vi "host.vi"() -> ()   [LabVIEW 2018]
uses:
  <vilib>/userdefined/High Color/nirio_resource_hc.ctl
  <instrlib>/niDCPower/nidcpower.llb/niDCPower Measurement Type.ctl
  <vilib>/FPGAPlugInAG/PXI-7953R/niLvFpga_Open_PXI-7953R.vi
  <vilib>/rvi/interface/common/dynamic/niFpgaDynamicAddResources.vi
  <vilib>/Utility/error.llb/Error Cluster From Error Code.vi
  <vilib>/rvi/errors/niLvFpgaAdjustHostInterfaceError.vi
  <vilib>/FPGAPlugInAG/Dynamic/niLvFpga_Close_Dynamic.vi
  <vilib>/rvi/interface/nirviOpenFPGA/nirviOpenFPGA.xnode
  FPGA Bitfiles/displayproj_FPGATarget_target_ybt1itgLS5Q.lvbitx
  <vilib>/rvi/interface/nirviReadWriteControl/nirviReadWriteControl.xnode
  <vilib>/rvi/interface/nirviCloseFPGA/nirviCloseFPGA.xnode
  NiFpgaLv.dll
  <vilib>/rvi/interface/Simulation/niFpgaSimulationCallBeginRW.vi
panel:
  out "LOS":bool
  out "FAULT":bool
  out "RX_DV/LOS":bool
  out "RX_ER/PRBS_PASS":bool
  in  "125MHZ_OE":bool
  in  "LOOPEN":bool
  in  "ENABLE":bool
  in  "LCKREFN":bool
  in  "PRBSEN":bool
  in  "Data":u8=24 format="%x"
  out "Array":bool[](array[boolean])=[FALSE, FALSE, FALSE, TRUE, FALSE, FALSE, FALSE, FALSE]
  out "IndxReadData":i32[](array[numeric])=[22, 24, 26, 28, 30, 32, 34, 36]
  in  "WRITE":bool
  out "DETECT":bool=TRUE
  in  "counterLowFreq":i32=120
  out "SDA_READED":u64=34637845889023
  out "size(s)":i32=46
  out "ACK_BOOL 2":bool=TRUE
  out "ACK_BOOL":bool=TRUE
  out "ACK 2":i32=41
  out "ACK":i32=23
  in  "TEST_EEPROM":bool=TRUE
  out "SPI_READY":bool=TRUE
  out "Vdd_Voltage, V 2":dbl=0.0007584113885058215 caption="V" format="%_3g"
  out "Vdd_Current, mA 2":dbl=-0.0058870491630167495 caption="mA" format="%_2g"
  in  "output enabled 2":bool caption="output enabled"
  in  "output enabled":bool
  out "Vdd_Current, mA":dbl=0.00018186713296160315 caption="mA" format="%_2g"
  out "Vdd_Voltage, V":dbl=-0.00013918231455023835 caption="V" format="%_3g"
  in  "Vdd":refnum<k15>="PXI1Slot2"
  in  "Tab Control":enum32{"Чтение EEPROM", "Проверка EEPROM"}(tab)=enum."Проверка EEPROM"
  in  "EEPROM_writePath":path caption="Путь для записи EEPROM"
  in  "EEPROM_checkPath":path caption="Путь для проверки EEPROM"
  out "REG_ERROR":i32
  out "Error List":string
  in  "FPGA name":T1="PXI1Slot5" caption="RIO Device"
  in  "Start":bool
  in  "Comand":bool
  in  "stop":bool=TRUE
  # "Ch2"
  # "Ch1"
  # "Запись/Чтение"
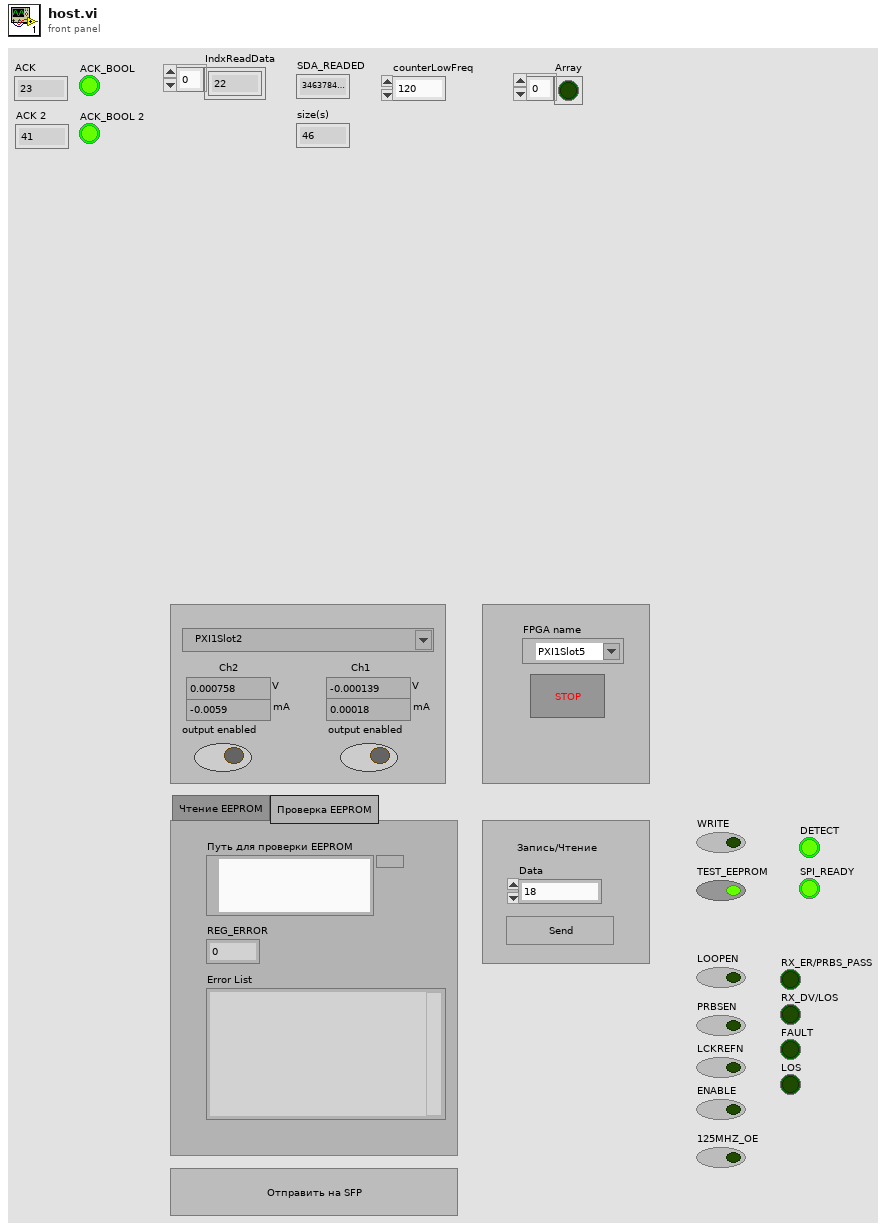
[diagram p1: front panel]
types:
  T1 = typedef "nirio_resource_hc.ctl" = tag
  T2 = enum16{"open", "replace", "create", "open or create", "replace or create", "replace or create with confirmation"}
  T3 = typedef "niDCPower Measurement Type.ctl" = i32
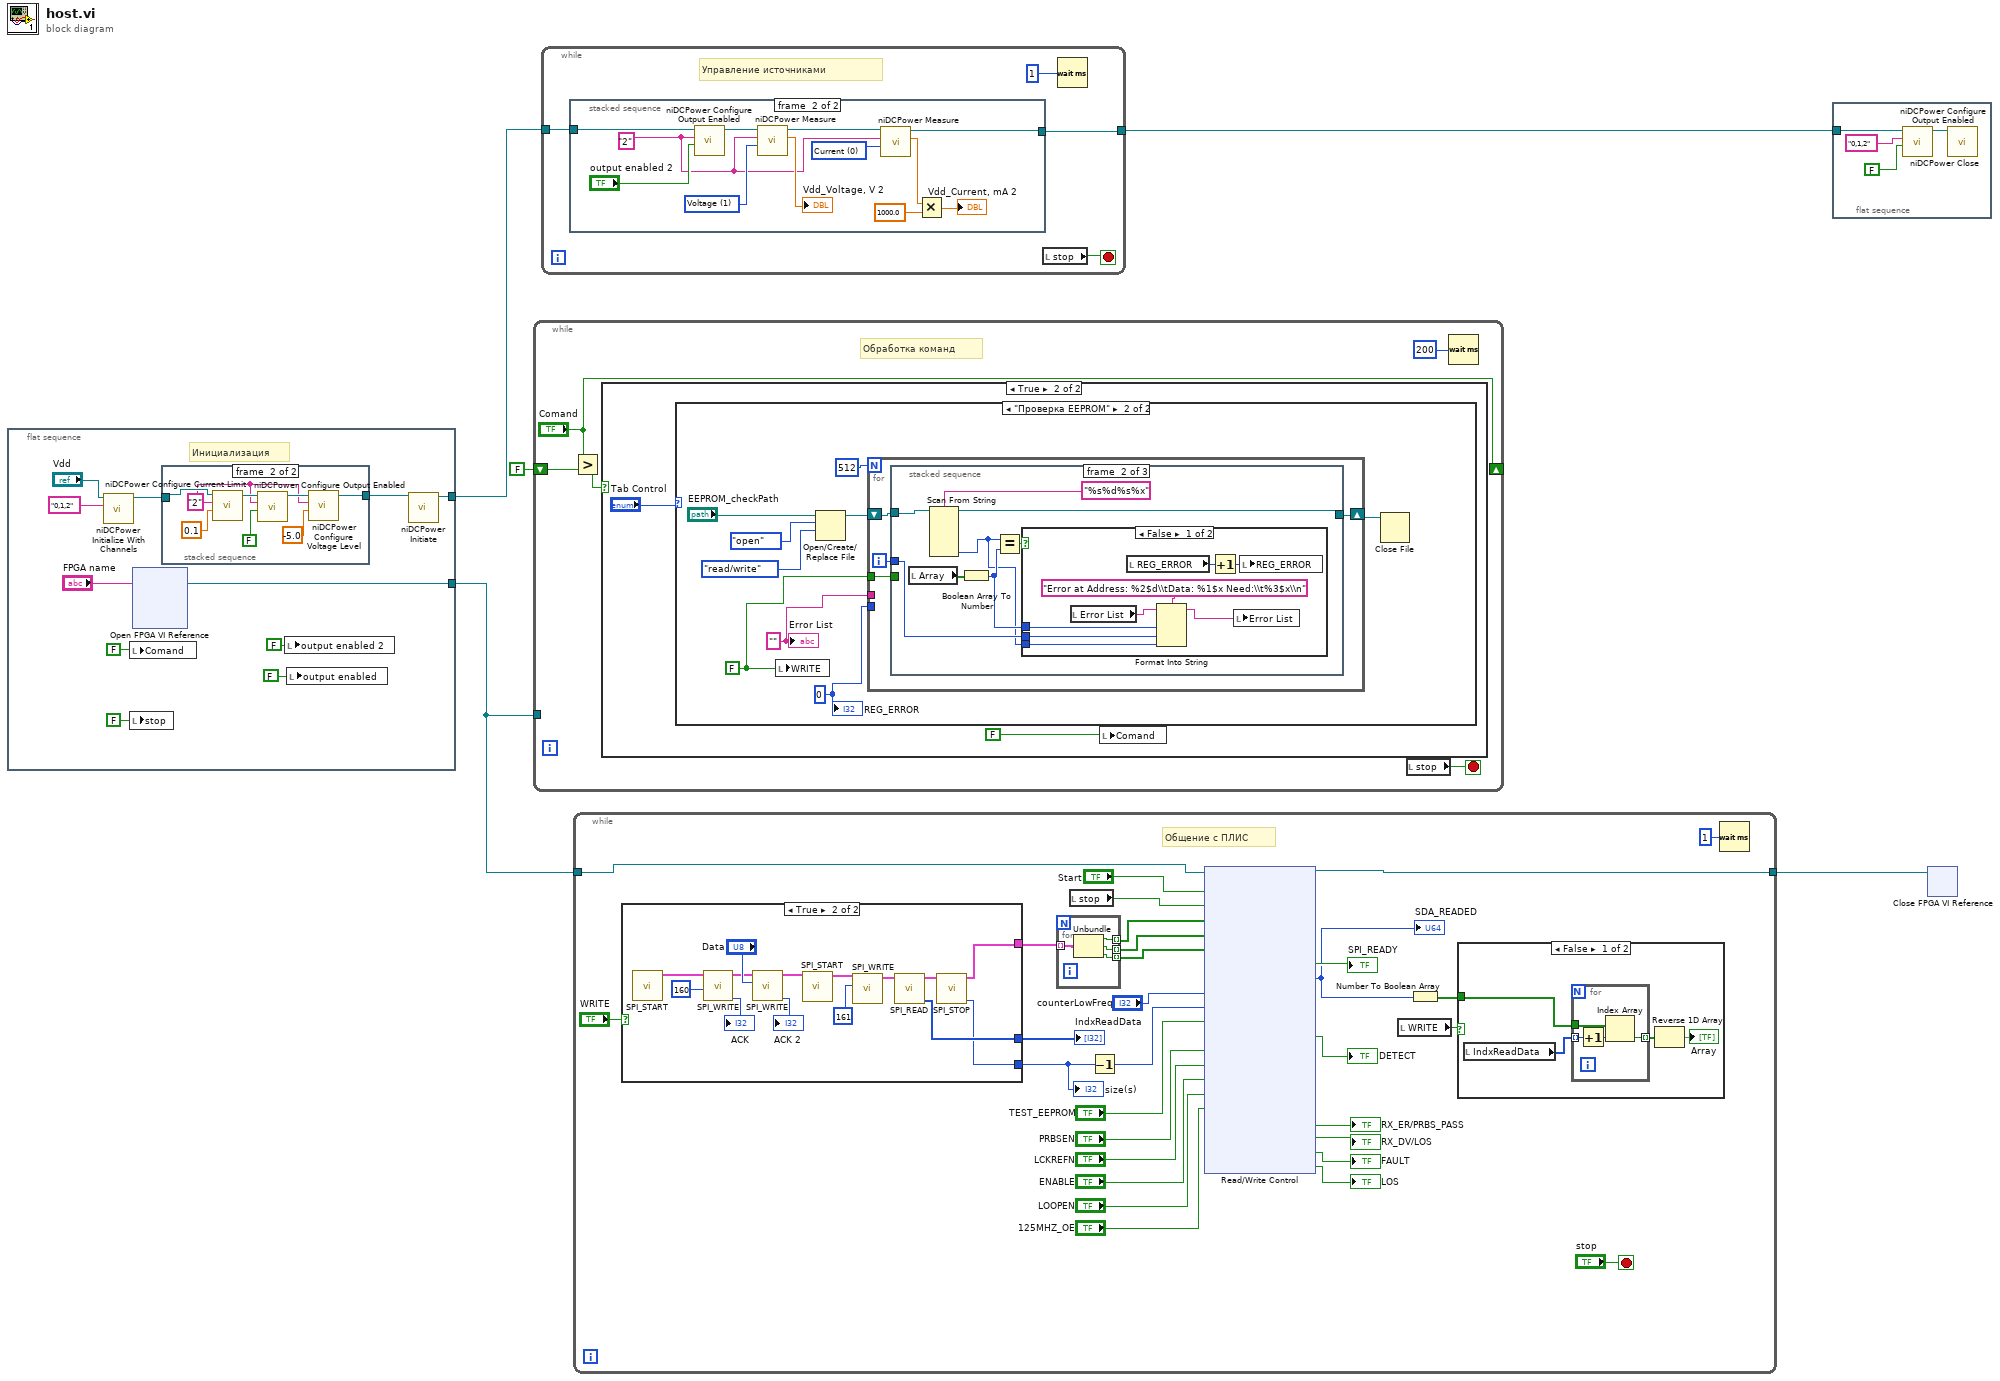
[diagram p0: block diagram]
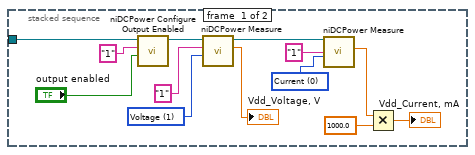
[diagram p2: hidden frame]
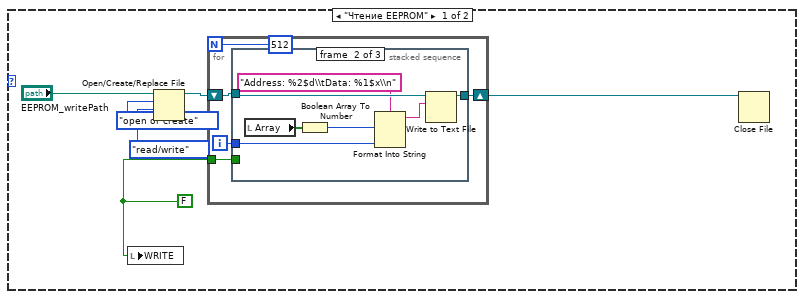
[diagram p4: hidden frame]
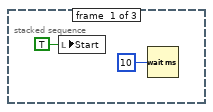
[diagram p5: hidden frame]
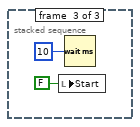
[diagram p6: hidden frame]
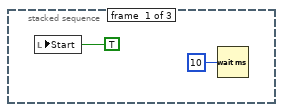
[diagram p7: hidden frame]
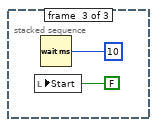
[diagram p9: hidden frame]
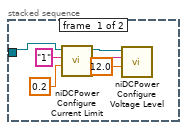
[diagram p10: hidden frame]
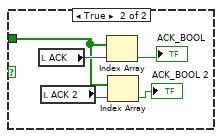
[diagram p11: hidden frame]
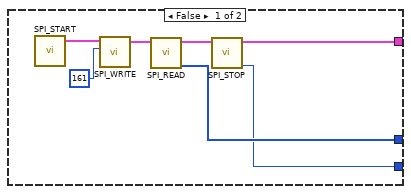
[diagram p12: hidden frame]
diagram:
  n1 = flat-sequence {
    tunnel: [w16] -> w4
    tunnel: [w8] -> w2
    frame #0 {
      # "Инициализация"
      n2 = call <instrlib>:"niDCPower Initialize With Channels.vi"("channels"="0,1,2", "resource name"="Vdd") -> ("instrument handle out"=w10:refnum<k15>)  [unwired: 8 in, 1 out]
      n3 = local write "Comand"(FALSE ("Comand")) -> ()
      n4 = local write "stop"(FALSE ("stop")) -> ()
      n5 = xnode "Open FPGA VI Reference"("resource name"="FPGA name") -> ("FPGA VI Reference Out"=w16:refnum<k20>)  [unwired: 1 in, 1 out]
      n6 = stacked-sequence {
        tunnel: [_ w27] -> w11
        tunnel: w10 -> [w20 w28]
        frame #0 {
          w18 = "1" ("channel name")
          n7 = call <instrlib>:"niDCPower Configure Current Limit.vi"("current limit"=0.2 ("current limit Vdd"), "channel name"=w18, "instrument handle"=w20) -> ("instrument handle out"=w19:refnum<k15>)  [unwired: 7 in, 1 out]
          n8 = call <instrlib>:"niDCPower Configure Voltage Level.vi"("voltage level"=12.0, "channel name"=w18, "instrument handle"=w19) -> ()  [unwired: 7 in, 2 out]
        }
        frame #1 {
          w24 = "2" ("channel name")
          n9 = call <instrlib>:"niDCPower Configure Current Limit.vi"("current limit"=0.1 ("current limit Vdd"), "channel name"=w24, "instrument handle"=w28) -> ("instrument handle out"=w25:refnum<k15>)  [unwired: 7 in, 1 out]
          n10 = call <instrlib>:"niDCPower Configure Output Enabled.vi"("output enabled"=FALSE, "channel name"=w24, "instrument handle"=w25) -> ("instrument handle out"=w26:refnum<k15>)  [unwired: 7 in, 1 out]
          n11 = call <instrlib>:"niDCPower Configure Voltage Level.vi"("voltage level"=-5.0, "channel name"=w24, "instrument handle"=w26) -> ("instrument handle out"=w27:refnum<k15>)  [unwired: 7 in, 1 out]
        }
      }
      n12 = local write "output enabled 2"(FALSE ("output enabled")) -> ()
      n13 = local write "output enabled"(FALSE ("output enabled")) -> ()
      n14 = call <instrlib>:"niDCPower Initiate.vi"("instrument handle"=w11) -> ("instrument handle out"=w8:refnum<k15>)  [unwired: 9 in, 1 out]
    }
  }
  n15 = while {
    tunnel: w4 -> [_]
    shift-right: ["Comand"] -> _
    shift-left: FALSE ("Comand") -> [w30]
    stop <- w34 stop-if-true
    # "Обработка команд"
    n16 = Greater?(x="Comand", y=w30) -> (0:w32:bool)
    n17 = case shown="True" w32 {
      frame False {
      }
      frame True {
        n18 = case shown="\"Проверка EEPROM\"" "Tab Control" {
          frame "Чтение EEPROM" {
            w38 = FALSE ("WRITE")
            n19 = local write "WRITE"(w38) -> ()
            n20 = Open/Create/Replace File(file path (use dialog)="EEPROM_writePath", operation (0:open)=T2."open or create", access (0:read/write)=enum16{"read/write", "read-only", "write-only"}."read/write") -> (refnum out=w40:refnum<file>)  [unwired: 3 in, 2 out]
            n21 = for {
              N: 512 -> [_]
              tunnel: w38 -> [w45]
              shift-right: [w46] -> w39
              shift-left: w40 -> [w47]
              i -> [w44]
              n22 = stacked-sequence {
                tunnel: w47 -> [_ w56 _]
                tunnel: [_ w55 _] -> w46
                tunnel: w45 -> [_ _ _]
                tunnel: w44 -> [_ w52 _]
                frame #0 {
                  n23 = local write "Start"(TRUE ("Start")) -> ()
                  n24 = Wait (ms)(milliseconds to wait=u32 10) -> ()  [unwired: 1 out]
                }
                frame #1 {
                  n25 = local read "Array"() -> (w54:bool[])
                  n26 = Boolean Array To Number(Boolean array=w54) -> (number=w53:u32)
                  n27 = Format Into String(format string="Address: %2$d\\tData: %1$x\\n", w53, w52) -> (resulting string=w51:string)  [unwired: 2 in, 1 out]
                  n28 = Write to Text File(file (use dialog)=w56, text=w51) -> (refnum out=w55:refnum<file>)  [unwired: 2 in, 2 out]
                }
                frame #2 {
                  n29 = local write "Start"(FALSE ("Start")) -> ()
                  n30 = Wait (ms)(milliseconds to wait=u32 10) -> ()  [unwired: 1 out]
                }
              }
            }
            n31 = Close File(refnum=w39) -> ()  [unwired: 1 in, 2 out]
          }
          frame "Проверка EEPROM" {
            w59 = "" ("String")
            w60 = 0 ("REG_ERROR")
            w62 = FALSE ("WRITE")
            n32 = local write "WRITE"(w62) -> ()
            n33 = Open/Create/Replace File(file path (use dialog)="EEPROM_checkPath", operation (0:open)=T2."open", access (0:read/write)=enum16{"read/write", "read-only", "write-only"}."read/write") -> (refnum out=w64:refnum<file>)  [unwired: 3 in, 2 out]
            n34 = for {
              N: 512 -> [_]
              tunnel: w62 -> [w69]
              shift-right: [w70] -> w63
              shift-left: w64 -> [w71]
              tunnel: w60 -> [_]
              tunnel: w59 -> [_]
              i -> [w68]
              n35 = stacked-sequence {
                tunnel: w71 -> [_ w79 _]
                tunnel: [_ w78 _] -> w70
                tunnel: w69 -> [_ _ _]
                tunnel: w68 -> [_ w75 _]
                frame #0 {
                  n36 = local write "Start"(TRUE ("Start")) -> ()
                  n37 = Wait (ms)(milliseconds to wait=u32 10) -> ()  [unwired: 1 out]
                }
                frame #1 {
                  n38 = local read "Array"() -> (w81:bool[])
                  n39 = Scan From String("%s%d%s%x" ("format string"), w79) -> (w78:refnum<file>, output 4=w74:u32)  [unwired: 8 in, 1 out]
                  n40 = Boolean Array To Number(Boolean array=w81) -> (number=w76:u32)
                  n41 = Equal?(x=w74, y=w76) -> (x = y?=w77:bool)
                  n42 = case shown="False" w77 {
                    tunnel: w76 -> [w87 _]
                    tunnel: w75 -> [w86 _]
                    tunnel: w74 -> [w82 _]
                    frame False {
                      n43 = local read "Error List"() -> (w83:string)
                      n44 = local read "REG_ERROR"() -> (w89:i32)
                      n45 = Format Into String(format string="Error at Address: %2$d\\tData: %1$x Need:\\t%3$x\\n", initial string=w83, w87, w86, w82) -> (resulting string=w84:string)  [unwired: 1 in, 1 out]
                      n46 = Increment(x=w89) -> (x+1=w88:i32)
                      n47 = local write "Error List"(w84) -> ()
                      n48 = local write "REG_ERROR"(w88) -> ()
                    }
                    frame True {
                    }
                  }
                }
                frame #2 {
                  n49 = local write "Start"(FALSE ("Start")) -> ()
                  n50 = Wait (ms)(milliseconds to wait=u32 10) -> ()  [unwired: 1 out]
                }
              }
            }
            n51 = Close File(refnum=w63) -> ()  [unwired: 1 in, 2 out]
            "REG_ERROR" <- w60
            "Error List" <- w59
          }
        }
        n52 = local write "Comand"(FALSE ("Comand")) -> ()
      }
    }
    n53 = local read "stop"() -> (w34:bool)
    n54 = Wait (ms)(milliseconds to wait=u32 200) -> ()  [unwired: 1 out]
  }
  n55 = while {
    tunnel: [w92] -> w3
    tunnel: w2 -> [w94]
    stop <- w95 stop-if-true
    # "Управление источниками"
    n56 = stacked-sequence {
      tunnel: w94 -> [w96 w111]
      tunnel: [_ w109] -> w92
      frame #0 {
        w103 = T3 0 items=["Current", "Voltage"] ("measurement type")
        w101 = T3 1 items=["Current", "Voltage"] ("measurement type")
        n57 = call <instrlib>:"niDCPower Configure Output Enabled.vi"("output enabled"="output enabled", "channel name"="1", "instrument handle"=w96) -> ("instrument handle out"=w105:refnum<k15>)  [unwired: 7 in, 1 out]
        n58 = call <instrlib>:"niDCPower Measure.vi"("measurement type"=w101, "channel name"="1", "instrument handle"=w105) -> ("measurement"=→"Vdd_Voltage, V":dbl, "instrument handle out"=w106:refnum<k15>)  [unwired: 6 in, 1 out]
        n59 = call <instrlib>:"niDCPower Measure.vi"("measurement type"=w103, "channel name"="1", "instrument handle"=w106) -> ("measurement"=w107:dbl)  [unwired: 6 in, 2 out]
        n60 = Multiply(x=w107, y=1000.0) -> (x*y=→"Vdd_Current, mA":dbl)
      }
      frame #1 {
        w116 = T3 0 items=["Current", "Voltage"] ("measurement type")
        w115 = T3 1 items=["Current", "Voltage"] ("measurement type")
        w110 = "2" ("channel name")
        n61 = call <instrlib>:"niDCPower Configure Output Enabled.vi"("output enabled"="output enabled 2", "channel name"=w110, "instrument handle"=w111) -> ("instrument handle out"=w117:refnum<k15>)  [unwired: 7 in, 1 out]
        n62 = call <instrlib>:"niDCPower Measure.vi"("measurement type"=w115, "channel name"=w110, "instrument handle"=w117) -> ("measurement"=→"Vdd_Voltage, V 2":dbl, "instrument handle out"=w118:refnum<k15>)  [unwired: 6 in, 1 out]
        n63 = call <instrlib>:"niDCPower Measure.vi"("measurement type"=w116, "channel name"=w110, "instrument handle"=w118) -> ("measurement"=w119:dbl, "instrument handle out"=w109:refnum<k15>)  [unwired: 6 in, 1 out]
        n64 = Multiply(x=w119, y=1000.0) -> (x*y=→"Vdd_Current, mA 2":dbl)
      }
    }
    n65 = local read "stop"() -> (w95:bool)
    n66 = Wait (ms)(milliseconds to wait=u32 1) -> ()  [unwired: 1 out]
  }
  n67 = while {
    tunnel: w4 -> [w149]
    tunnel: [w148] -> w5
    stop <- "stop" stop-if-true
    # "Общение с ПЛИС"
    n68 = case shown="True" "WRITE" {
      tunnel: [w168 w175] -> w131
      tunnel: [w170 w177] -> w136
      tunnel: [w169 w176] -> w135
      frame False {
        n69 = call "SPI_START.vi"() -> ("cluster out"=w173:cluster{bool, bool, bool}[])  [unwired: 9 in, 1 out]
        n70 = call "SPI_WRITE.vi"("cluster in"=w173, "Data"=u8 161) -> ("cluster out"=w172:cluster{bool, bool, bool}[])  [unwired: 6 in, 2 out]
        n71 = call "SPI_READ.vi"("cluster in"=w172) -> ("IndxReadData"=w170:i32[], "cluster out"=w171:cluster{bool, bool, bool}[])  [unwired: 8 in, 1 out]
        n72 = call "SPI_STOP.vi"("cluster in"=w171) -> ("size(s)"=w168:i32, "cluster out"=w169:cluster{bool, bool, bool}[])  [unwired: 6 in]
      }
      frame True {
        n73 = call "SPI_START.vi"() -> ("cluster out"=w183:cluster{bool, bool, bool}[])  [unwired: 9 in, 1 out]
        n74 = call "SPI_WRITE.vi"("cluster in"=w183, "Data"=u8 160) -> ("cluster out"=w182:cluster{bool, bool, bool}[], "ACK"=→"ACK":i32)  [unwired: 6 in, 1 out]
        n75 = call "SPI_WRITE.vi"("cluster in"=w182, "Data"="Data") -> ("cluster out"=w181:cluster{bool, bool, bool}[], "ACK"=→"ACK 2":i32)  [unwired: 6 in, 1 out]
        n76 = call "SPI_START.vi"("cluster in"=w181) -> ("cluster out"=w180:cluster{bool, bool, bool}[])  [unwired: 8 in, 1 out]
        n77 = call "SPI_WRITE.vi"("cluster in"=w180, "Data"=u8 161) -> ("cluster out"=w179:cluster{bool, bool, bool}[])  [unwired: 6 in, 2 out]
        n78 = call "SPI_READ.vi"("cluster in"=w179) -> ("IndxReadData"=w177:i32[], "cluster out"=w178:cluster{bool, bool, bool}[])  [unwired: 8 in, 1 out]
        n79 = call "SPI_STOP.vi"("cluster in"=w178) -> ("size(s)"=w175:i32, "cluster out"=w176:cluster{bool, bool, bool}[])  [unwired: 6 in]
      }
    }
    "IndxReadData" <- w136
    "size(s)" <- w131
    n80 = for {
      tunnel: w135 -> [w154] mode=indexing
      tunnel: [w153] -> w134 mode=indexing
      tunnel: [w152] -> w133 mode=indexing
      tunnel: [w151] -> w132 mode=indexing
      n81 = Unbundle(w154) -> (w153:bool, w152:bool, w151:bool)
    }
    n82 = local read "stop"() -> (w145:bool)
    n83 = Decrement(x=w131) -> (x-1=w130:i32)
    n84 = xnode "Read/Write Control"("FPGA VI Reference In"=w149, "Start"="Start", "stop"=w145, "SDA_array"=w134, "SCL_array"=w133, "PFI_WE_array"=w132, "counterLowFreq"="counterLowFreq", "SPI_END"=w130, "TEST_EEPROM"="TEST_EEPROM", "PRBSEN"="PRBSEN", "LCKREFN"="LCKREFN", "ENABLE"="ENABLE", "LOOPEN"="LOOPEN", "125MHZ_OE"="125MHZ_OE") -> ("FPGA VI Reference Out"=w148:refnum<k20>, "SPI_READY"=→"SPI_READY":bool, "SDA_READED"=w141:u64, "DETECT"=→"DETECT":bool, "RX_ER/PRBS_PASS"=→"RX_ER/PRBS_PASS":bool, "RX_DV/LOS"=→"RX_DV/LOS":bool, "FAULT"=→"FAULT":bool, "LOS"=→"LOS":bool)  [unwired: 1 in, 1 out]
    "SDA_READED" <- w141
    n85 = local read "WRITE"() -> (w137:bool)
    n86 = Number To Boolean Array(number=w141) -> (Boolean array=w140:bool[])
    n87 = case shown="False" w137 {
      tunnel: w140 -> [w158 w165]
      frame False {
        n88 = local read "IndxReadData"() -> (w157:i32[])
        n89 = for {
          tunnel: w158 -> [w162]
          tunnel: w157 -> [w160] mode=indexing
          tunnel: [w161] -> w156 mode=indexing
          n90 = Increment(x=w160) -> (x+1=w159:i32)
          n91 = Index Array(array=w162, index=w159) -> (element=w161:bool)
        }
        n92 = Reverse 1D Array(array=w156) -> (reversed array=→"Array":bool[])
      }
      frame True {
        n93 = local read "ACK"() -> (w167:i32)
        n94 = local read "ACK 2"() -> (w166:i32)
        n95 = Index Array(array=w165, index=w167) -> (element=→"ACK_BOOL":bool)
        n96 = Index Array(array=w165, index=w166) -> (element=→"ACK_BOOL 2":bool)
      }
    }
    n97 = Wait (ms)(milliseconds to wait=u32 1) -> ()  [unwired: 1 out]
  }
  n98 = flat-sequence {
    tunnel: w3 -> [w192]
    frame #0 {
      n99 = call <instrlib>:"niDCPower Configure Output Enabled.vi"("output enabled"=FALSE, "channel name"="0,1,2", "instrument handle"=w192) -> ("instrument handle out"=w190:refnum<k15>)  [unwired: 7 in, 1 out]
      n100 = call <instrlib>:"niDCPower Close.vi"("instrument handle"=w190) -> ()  [unwired: 10 in, 1 out]
    }
  }
  n101 = xnode "Close FPGA VI Reference"("FPGA VI Reference In"=w5) -> ()  [unwired: 1 in, 1 out]
